vi "Assemble fragments.vi"(2 "Numeric":i32, 3 "Array in":cluster{"data":u8[]}[](array[cluster])) -> (1 "Array out":u8[](array[numeric]))   [LabVIEW 2020, in "NI_Bytestream.lvlib" / "Bytestream.lvclass"]
uses:
  <vilib>/Array/Bytestream/Bytestream.lvclass
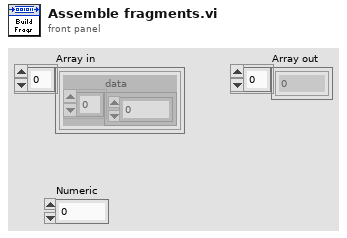
[diagram p1: front panel]
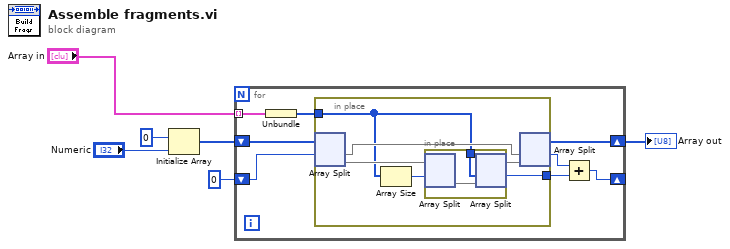
[diagram p0: block diagram]
diagram:
  n1 = Initialize Array(u8 0, "Numeric") -> (w3:u8[])
  n2 = for {
    shift-right: [w10] -> w6
    shift-left: w3 -> [w13]
    tunnel: "Array in" -> [w14] mode=indexing
    shift-right: [w7] -> _
    shift-left: 0 -> [w12]
    n3 = Unbundle(w14) -> ("data"=w11:u8[])
    n4 = in-place {
      in-place-border: w11 -> [w17]
      in-place-border: [w15] -> w8
      n5 = in-place-split #1(w13, w12) -> (w19:u8[], w20:u8[])
      n6 = Array Size(array=w17) -> (size(s)=w16:i32)
      n7 = in-place {
        in-place-border: w17 -> [w21]
        n8 = in-place-split #2(w20, w16) -> (w22:u8[])  [unwired: 1 out]
        n9 = in-place-split #2(w21, w22) -> (w18:u8[], w15:i32)
      }
      n10 = in-place-split #1(w19, w18) -> (w10:u8[], w9:i32)
    }
    n11 = Add(x=w9, y=w8) -> (x+y=w7:i32)
  }
  "Array out" <- w6
